vi "linear_ramp_accel.vi"(10 "filter const (dx/dt)":dbl, 11 "input":dbl) -> (3 "output":dbl)   [LabVIEW 2015]
panel:
  # "dx is in input units\ndt is in seconds"
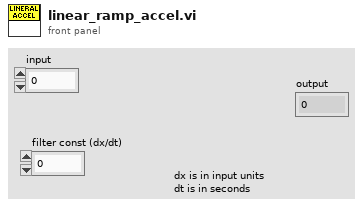
[diagram p1: front panel]
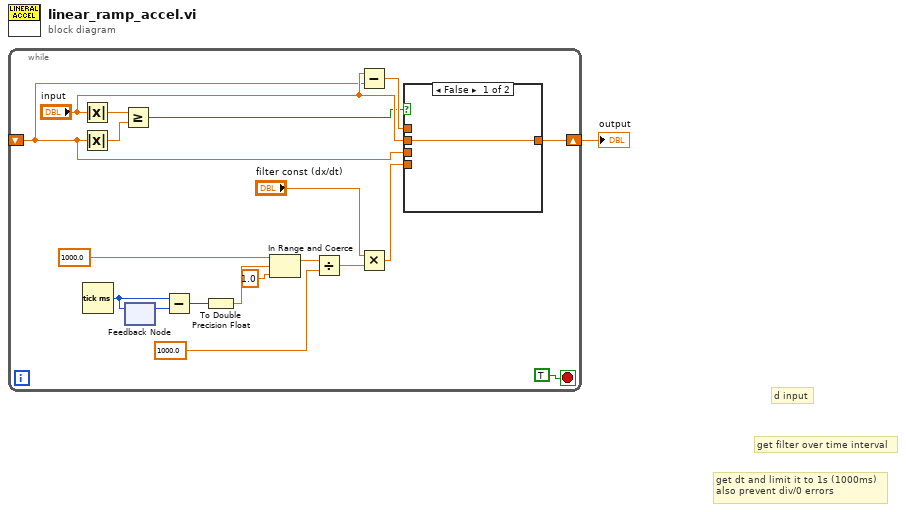
[diagram p0: block diagram]
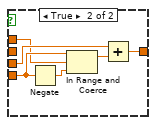
[diagram p2: hidden frame]
diagram:
  # "get filter over time interval"
  # "get dt and limit it to 1s (1000ms)\nalso prevent div/0 errors"
  # "d input"
  n1 = while {
    shift-right: [w9] -> w1
    shift-left: _ -> [w2]
    stop <- TRUE stop-if-true
    n2 = Absolute Value(x="input") -> (abs(x)=w4:dbl)
    n3 = Absolute Value(x=w2) -> (abs(x)=w5:dbl)
    n4 = Tick Count (ms)() -> (millisecond timer value=w19:u32)
    n5 = Greater Or Equal?(x=w4, y=w5) -> (x >= y?=w3:bool)
    n6 = feedback-in #1(w19) -> ()
    n7 = feedback #1() -> (w18:u32)  [unwired: 1 in]
    n8 = Subtract(x=w19, y=w18) -> (x-y=w17:u32)
    n9 = To Double Precision Float(number=w17) -> (double precision float=w16:dbl)
    n10 = In Range and Coerce(upper limit=1000.0, x=w16, lower limit=1.0) -> (coerced(x)=w12:dbl)  [unwired: 1 out]
    n11 = Divide(x=w12, y=1000.0) -> (x/y=w10:dbl)
    n12 = Subtract(x="input", y=w2) -> (x-y=w7:dbl)
    n13 = Multiply(x="filter const (dx/dt)", y=w10) -> (x*y=w8:dbl)
    n14 = case shown="False" w3 {
      tunnel: [w21 w25] -> w9
      tunnel: w8 -> [_ w24]
      tunnel: w2 -> [_ w23]
      tunnel: w7 -> [_ w22]
      tunnel: "input" -> [w21 _]
      frame False {
      }
      frame True {
        n15 = Negate(x=w24) -> (-x=w27:dbl)
        n16 = In Range and Coerce(upper limit=w24, x=w22, lower limit=w27) -> (coerced(x)=w26:dbl)  [unwired: 1 out]
        n17 = Add(x=w23, y=w26) -> (x+y=w25:dbl)
      }
    }
  }
  "output" <- w1
